vi "exportGraphsToPDF.vi"(7 "PatientID":string, 8 "error in (no error)":errorcluster, 9 "Type":string, 10 "Text":string, 11 "Folder":string) -> (0 "error out":errorcluster)   [LabVIEW 2013, in "main.lvlib"]
uses:
  main.lvlib
  <userlib>/Exaprom PDF/Controls/Header or Footer  Text cluster.ctl
  <userlib>/Exaprom PDF/Controls/H F Alignment.ctl
  <userlib>/Exaprom PDF/Controls/Font cluster.ctl
  <userlib>/Exaprom PDF/Controls/Font size.ctl
  <userlib>/Exaprom PDF/Controls/Font color.ctl
  <userlib>/Exaprom PDF/Controls/Header or Footer.ctl
  <userlib>/Exaprom PDF/Controls/Page setup.ctl
  <userlib>/Exaprom PDF/Controls/Page size.ctl
  <userlib>/Exaprom PDF/Controls/Page Orientation.ctl
  <userlib>/Exaprom PDF/Controls/Page Layout Custom.ctl
  <userlib>/Exaprom PDF/Controls/Page margins.ctl
  <userlib>/Exaprom PDF/Controls/PDF Details.ctl
  <userlib>/Exaprom PDF/Controls/Paragraphe cluster.ctl
  <userlib>/Exaprom PDF/Controls/Texte alignement.ctl
  <userlib>/Exaprom PDF/Controls/Line spacing.ctl
  Globals/DataPathGlobalVariable.vi
  <userlib>/Exaprom PDF/VIs/Low level/Header, Footer and Watermark Low level/Append Text HF.vi
  <userlib>/Exaprom PDF/VIs/Text/Append Paragraph.vi
panel:
  in  "Blue 2":refnum<vi>
  out "Blue":dbl[][](graph)
  out "Red":dbl[][](graph)
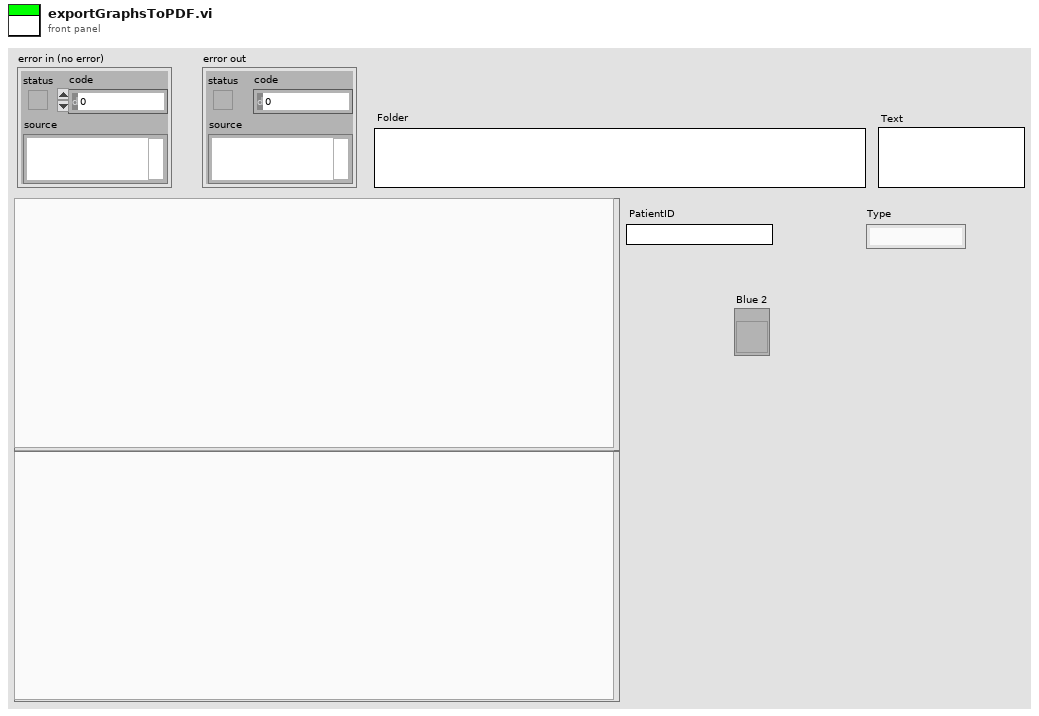
[diagram p1: front panel]
types:
  T1 = typedef "PDF Details.ctl" = cluster{"Title":string, "Subject":string, "Keywords":string, "Author":string, "Creator":string}
  T2 = typedef "Page setup.ctl" = cluster{"Page Size":T3, "Orientation":T4, "Custom Layout":T5, "Margins":T6}
  T3 = typedef "Page size.ctl" = i32
  T4 = typedef "Page Orientation.ctl" = enum16{"Portrait", "Landscape"}
  T5 = typedef "Page Layout Custom.ctl" = cluster{"Width":sgl, "Height":sgl}
  T6 = typedef "Page margins.ctl" = cluster{"Left":sgl, "Right":sgl, "Top":sgl, "Bottom":sgl}
  T7 = typedef "H F Alignment.ctl" = enum16{"LEFT - top", "LEFT - middle", "LEFT - bottom", "CENTER - top", "CENTER - middle", "CENTER - bottom", "RIGHT - top", "RIGHT - middle", "RIGHT - bottom", ""}
  T8 = typedef "Header or Footer.ctl" = enum16{"Header", "Footer"}
  T9 = typedef "Header or Footer  Text cluster.ctl" = cluster{"Start at page":i32, "H/F Alignment":T7, "Text":string, "Font":T10, "Link":string}
  T10 = typedef "Font cluster.ctl" = cluster{"Name":string, "Size":T11, "Color":T12, "Style":cluster{"Bold":bool, "Italic":bool, "Underline":bool, "Strikeout":bool}}
  T11 = typedef "Font size.ctl" = sgl
  T12 = typedef "Font color.ctl" = u32
  T13 = typedef "Unit.ctl" = enum16{"inch", "mm"}
  T14 = typedef "Paragraphe cluster.ctl" = cluster{" Aligment":T15, "Line spacing":T16}
  T15 = typedef "Texte alignement.ctl" = enum16{"Select", "CENTER", "JUSTIFY", "LEFT", "RIGHT"}
  T16 = typedef "Line spacing.ctl" = enum16{"Select", "1.0", "1.5", "2.0"}
  T17 = typedef "Page dimensions.ctl" = cluster{"Start at page":i32, "Orientation":T4, "widht":sgl, "height":sgl, "Margin left":sgl, "Margin right":sgl, "Margin top":sgl, "Margin bottom":sgl}
  T18 = typedef "Image or Table Caption.ctl" = cluster{"Caption":string, "Separator":string, "Position":enum16{"Above", "Below"}}
  T19 = typedef "Header Footer [ ].ctl" = T20[]
  T20 = typedef "Header Footer cluster.ctl" = cluster{"Start page":i32, "Type":T21, "Alignment":T22, "Vertical Alignement":T23, "Image (%)":sgl, "Page #":T24, "Text":string, "Path":string, "Font":T10, "Font refnum":refnum<k24>, "Line":cluster{"Line":T25, "Thickness (points)":sgl, "Colour":T12}}
  T21 = typedef "Header Footer Type.ctl" = enum16{"Select", "Text", "Text + hyperlink", "Page number", "Image", "Image + hyperlink"}
  T22 = typedef "Header footer horiz alignment.ctl" = enum16{"Left", "Center", "Right"}
  T23 = typedef "Cell Vertical alignment.ctl" = enum16{"TOP", "MIDDLE", "BOTTOM"}
  T24 = typedef "Page number.ctl" = cluster{"Text 1":string, "Text 2":string, "Text 3":string}
  T25 = typedef "Header Footer Line.ctl" = enum16{"No line", "Horizontal line"}
  T26 = typedef "Watermark cluster2.ctl" = cluster{"Show? (F)":bool, "Type":enum16{"Image", "Text"}, "Opacity (%)":sgl, "Rotate(°)":sgl, "Position":cluster{"Position":T27, "X":sgl, "Y":sgl}, "Image path":path, "Scaled(%)":sgl, "Image refnum":refnum<k24>, "Text":string, "Font":cluster{"Name":string, "Size":T11, "Color":T12}, "Font refnum":refnum<k24>, "Alignment":T22, "Automatic":bool}
  T27 = typedef "Watermark Position.ctl" = enum16{"Absolute", "Center (page)", "Center (text section)"}
  T28 = typedef "System Fonts.ctl" = cluster{"Font name [ ]":string[], "Font and file names [ ]":cluster{"Font name":string, "File name":string}[]}
  T29 = cluster{"Document":refnum<k24>, "Writer":refnum<k24>, "Default Font":refnum<k24>, "Default Font cluster":T10, "Path":path, "Unit (default = mm)":T13, "Paragraphe cluster":T14, "Pages dimensions [ ]":T17[], "Captions":cluster{"Image":T18, "Image counter":u16, "Table":T18, "Table counter":u16, "Font":T10}, "Header":T19, "Footer":T19, "Watermark ":T26, "Actual VI name":string, "System Fonts":T28}
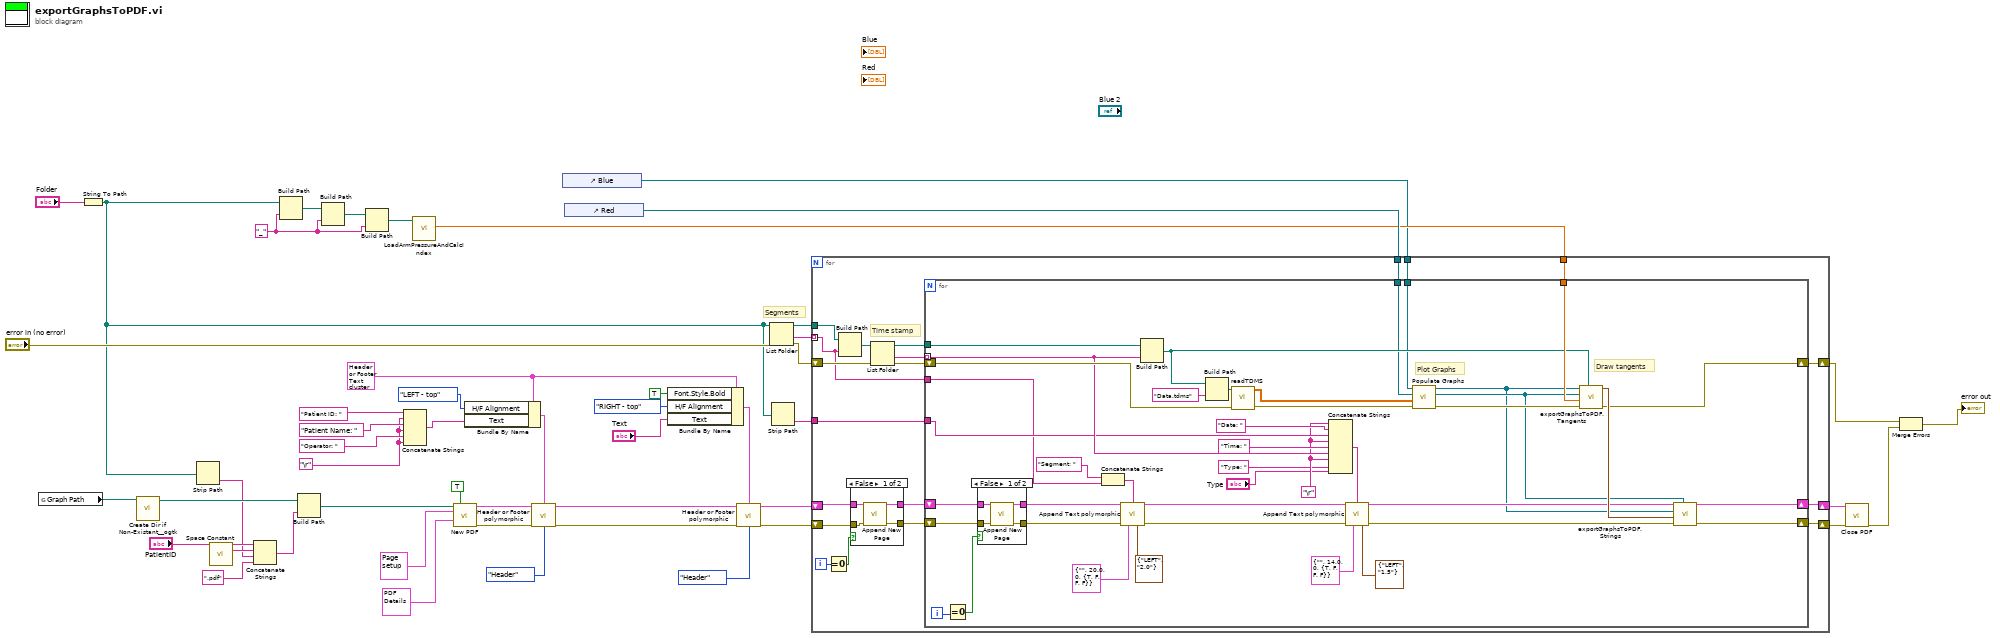
[diagram p0: block diagram]
diagram:
  w1 = "\r"
  w30 = T9 {"Start at page"=1, "H/F Alignment"=enum."LEFT - top", "Text"="", "Font"={"Name"="Helvetica", "Size"=12.0, "Color"=0, "Style"={"Bold"=FALSE, "Italic"=FALSE, "Underline"=FALSE, "Strikeout"=FALSE}}, "Link"=""} ("Header or footer")
  w37 = "_" ("name or relative path")
  # "Segments"
  n1 = global read "DataPathGlobalVariable.vi" "Graph Path"() -> (w6:path)
  n2 = String To Path(string="Folder") -> (path=w8:path)
  n3 = call <userlib>:"Create Dir if Non-Existant__ogtk.vi"("Directory Path"=w6) -> ("dup Directory Path"=w12:path)  [unwired: 8 in, 2 out]
  n4 = Strip Path(path=w8) -> (name=w10:string)  [unwired: 1 out]
  n5 = call <vilib>:"Space Constant.vi"() -> ("String"=w11:string)
  n6 = Concatenate Strings("PatientID", w11, w10, ".pdf" ("string")) -> (w15:string)
  n7 = Build Path(base path=w8, name or relative path=w37) -> (appended path=w39:path)
  n8 = Build Path(base path=w12, name or relative path=w15) -> (appended path=w14:path)
  n9 = Build Path(base path=w39, name or relative path=w37) -> (appended path=w38:path)
  n10 = Build Path(base path=w38, name or relative path=w37) -> (appended path=w36:path)
  n11 = Concatenate Strings("Patient ID: ", w1, "Patient Name: ", w1, "Operator: ", w1) -> (w23:string)
  n12 = call "LoadArmPressureAndCalcIndex.vi"("Path"=w36) -> ("Armpressure"=w21:dbl)  [unwired: 8 in, 2 out]
  n13 = call <userlib>:"New PDF.vi"("PDF Path"=w14, "Overwrite?"=TRUE, "Page Setup"=T2 {"Page Size"=11, "Orientation"=enum."Portrait", "Custom Layout"={"Width"=216.0, "Height"=279.0}, "Margins"={"Left"=25.0, "Right"=25.0, "Top"=25.0, "Bottom"=25.0}}, "PDF Details"=T1 {"Title"="", "Subject"="", "Keywords"="", "Author"="", "Creator"="Medimatic DM2000 Digital"}) -> ("PDF Report"=w43:T29, "error out"=w42:errorcluster)  [unwired: 10 in]
  n14 = Bundle By Name(cluster=w30, "H/F Alignment"=H_F_Alignment."LEFT - top", "Text"=w23) -> (w40:T9)
  n15 = call-poly <userlib>:"Header or Footer polymorphic.vi"("PDF Report IN"=w43, "Header or footer"=w40, "error in (no error)"=w42, "Position"=Header_or_Footer."Header") -> ("PDF Report OUT"=w35:T29, "error out"=w34:errorcluster)  [unwired: 10 in]
  n16 = control-ref of="Blue"() -> (w2:refnum<vi>)
  n17 = control-ref of="Red"() -> (w44:refnum<vi>)
  n18 = Bundle By Name(cluster=w30, "Font.Style.Bold"=TRUE, "H/F Alignment"=H_F_Alignment."RIGHT - top", "Text"="Text") -> (w27:T9)
  n19 = call-poly <userlib>:"Header or Footer polymorphic.vi"("PDF Report IN"=w35, "Header or footer"=w27, "error in (no error)"=w34, "Position"=Header_or_Footer."Header") -> ("PDF Report OUT"=w33:T29, "error out"=w32:errorcluster)  [unwired: 10 in]
  n20 = List Folder(path=w8, error in="error in (no error)") -> (path out=w48:path, folder names=w49:string[], error out=w47:errorcluster)  [unwired: 2 in, 1 out]
  n21 = Strip Path(path=w8) -> (name=w7:string)  [unwired: 1 out]
  n22 = for {
    tunnel: w49 -> [w52] mode=indexing
    tunnel: w48 -> [w69]
    tunnel: w44 -> [w66]
    tunnel: w2 -> [w65]
    tunnel: w21 -> [w64]
    shift-right: [w61] -> w3
    shift-left: w47 -> [w62]
    shift-right: [w59] -> w4
    shift-left: w32 -> [w57]
    shift-right: [w60] -> w5
    shift-left: w33 -> [w56]
    tunnel: w7 -> [w51]
    i -> [w58]
    # "Time stamp"
    n23 = Equal To 0?(x=w58) -> (x = 0?=w55:bool)
    n24 = Build Path(base path=w69, name or relative path=w52) -> (appended path=w70:path)
    n25 = case shown="False" w55 {
      tunnel: [w72 w76] -> w54
      tunnel: [w71 w75] -> w53
      tunnel: w57 -> [w74 w75]
      tunnel: w56 -> [w73 w76]
      frame False {
        n26 = call <userlib>:"Append New Page.vi"("PDF Report"=w73, "error in (no error)"=w74) -> ("PDF Report duplicate"=w72:T29, "error OUT"=w71:errorcluster)  [unwired: 12 in]
      }
      frame True {
      }
    }
    n27 = List Folder(path=w70, error in=w62) -> (path out=w68:path, folder names=w67:string[], error out=w63:errorcluster)  [unwired: 2 in, 1 out]
    n28 = for {
      tunnel: w68 -> [w116]
      tunnel: w67 -> [w101] mode=indexing
      tunnel: w66 -> [w83]
      tunnel: w65 -> [w82]
      tunnel: w64 -> [w115]
      shift-right: [w105] -> w61
      shift-left: w63 -> [w111]
      shift-right: [w108] -> w59
      shift-left: w53 -> [w95]
      shift-right: [w109] -> w60
      shift-left: w54 -> [w96]
      tunnel: w52 -> [w87]
      tunnel: w51 -> [w90]
      i -> [w104]
      w79 = "\r"
      # "Draw tangents"
      # "Plot Graphs"
      n29 = Equal To 0?(x=w104) -> (x = 0?=w92:bool)
      n30 = case shown="False" w92 {
        tunnel: [w120 w122] -> w93
        tunnel: [w119 w121] -> w94
        tunnel: w96 -> [w118 w122]
        tunnel: w95 -> [w117 w121]
        frame False {
          n31 = call <userlib>:"Append New Page.vi"("PDF Report"=w118, "error in (no error)"=w117) -> ("PDF Report duplicate"=w120:T29, "error OUT"=w119:errorcluster)  [unwired: 12 in]
        }
        frame True {
        }
      }
      n32 = Concatenate Strings("Segment: ", w87) -> (w89:string)
      n33 = call-poly <userlib>:"Append Text polymorphic.vi"("PDF Report"=w93, "Text"=w89, "error in (no error)"=w94, "Font"=T10 {"Name"="", "Size"=20.0, "Color"=0, "Style"={"Bold"=TRUE, "Italic"=FALSE, "Underline"=FALSE, "Strikeout"=FALSE}}, "Paragraph properties"=T14 {" Aligment"=enum."LEFT", "Line spacing"=enum."2.0"}) -> ("PDF Report duplicate"=w81:T29, "error out"=w80:errorcluster)  [unwired: 9 in]
      n34 = Build Path(base path=w116, name or relative path=w101) -> (appended path=w114:path)
      n35 = Build Path(base path=w114, name or relative path="Data.tdms") -> (appended path=w112:path)
      n36 = call "readTDMS.vi"("error in (no error)"=w111, "Path Out"=w112) -> ("error out"=w86:errorcluster, "Array"=w85:dbl[][])  [unwired: 8 in]
      n37 = Concatenate Strings(w79, "Date: ", w90, w79, "Time: " ("string"), w101, w79, "Type: ", "Type") -> (w100:string)
      n38 = call-poly <userlib>:"Append Text polymorphic.vi"("PDF Report"=w81, "Text"=w100, "error in (no error)"=w80, "Font"=T10 {"Name"="", "Size"=14.0, "Color"=0, "Style"={"Bold"=TRUE, "Italic"=FALSE, "Underline"=FALSE, "Strikeout"=FALSE}}, "Paragraph properties"=T14 {" Aligment"=enum."LEFT", "Line spacing"=enum."1.5"}) -> ("PDF Report duplicate"=w106:T29, "error out"=w107:errorcluster)  [unwired: 9 in]
      n39 = call "Populate Graphs.vi"("error in (no error)"=w86, "Array"=w85, "Red"=w83, "Blue"=w82) -> ("error out"=w84:errorcluster)  [unwired: 7 in]
      n40 = call "exportGraphsToPDF.Tangents.vi"("path"=w114, "error in (no error)"=w84, "Armpressure"=w115, "Red Graph"=w83, "Blue Graph"=w82) -> ("error out"=w105:errorcluster, "output cluster"=w110:cluster{dbl, dbl, dbl, dbl})  [unwired: 5 in]
      n41 = call "exportGraphsToPDF.Strings.vi"("Red"=w83, "error in (no error)"=w107, "Input Cluster"=w110, "Blue"=w82, "PDF Report duplicate"=w106) -> ("error out"=w108:errorcluster, "PDF Report OUT"=w109:T29)  [unwired: 5 in]
    }
  }
  n42 = call <userlib>:"Close PDF.vi"("PDF Report"=w5, "error in (no error)"=w4) -> ("error out"=w45:errorcluster)  [unwired: 12 in, 1 out]
  n43 = Merge Errors(w3, w45) -> (→"error out":errorcluster)
